vi "DFD Validate Obj.vi"   [LabVIEW 2017, in "NI_DigFilterLicensed.lvlib"]
doc: "Validates a filter based on the information saved in the input object. You can use this polymorphic VI to validate a filter or a multirate filter. The filter you wire to <B>filter in</B> determines the polymorphic instance."
uses:
  <vilib>/addons/Digital Filter Design/NI_DigFilterLicensed.lvlib
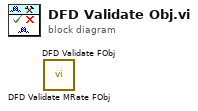
[diagram p0: block diagram]
diagram:
  n1 = call <vilib>:"DFD Validate MRate FObj.vi"() -> ()  [unwired: 8 in, 4 out]
  n2 = call <vilib>:"DFD Validate FObj.vi"() -> ()  [unwired: 9 in, 3 out]
